vi "Constants.vi"() -> ()   [LabVIEW 2018, in "TestCD Shared.lvlib"]
doc: "Use this Global VI to access the GUIDs assigned to the page resources of the Custom Device."
uses:
  TestCD Shared.lvlib
panel:
  in  "Tab Control":enum32{"GUIDS", "Constants", "Properties"}(tab)
  in  "TestCD":string="cdbebeb8-7607-4c68-9659-8a019886b0ce"
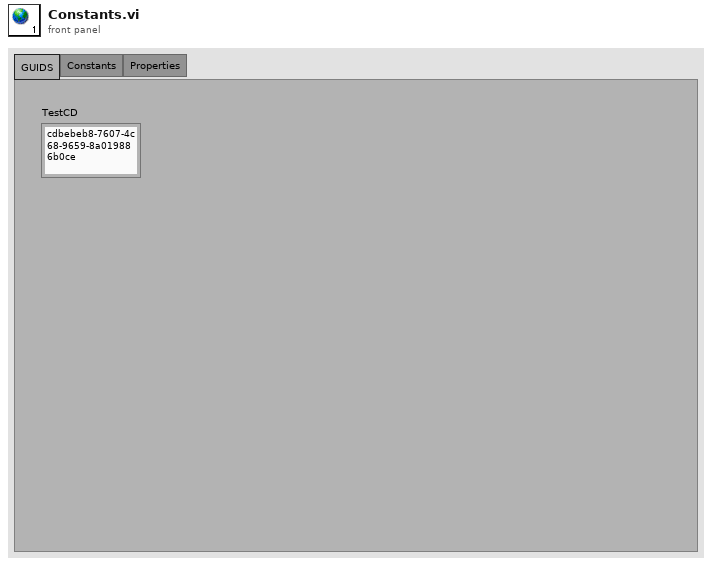
[diagram p1: front panel]
diagram:
